vi "CalVEIN Main FRANK TEST.vi"() -> ()   [LabVIEW 2016]
uses:
  Type Defs/Sensor Data.ctl
  Type Defs/Boxcar.ctl
panel:
  out "1st loop":i32
  out "45% 2":string="31.00 °C"
  out "45%":string="31.10 °C"
  in  "Box cooler":bool
  out "NewVal":bool
  out "Ready To Fire Flag":bool
  out "Firing State":string[](array[string])=["System Is Not Armed", "", "", "", "", " "]
  in  "Arm Flag":bool
  in  "Sample Rate (secs)":u32=1000
  out "Burn Time\nCountdown (secs)":string="0.00"
  out "Boxcar Data":T1={"AI Sensor Data"={"Sensor Array"=[{"Description"="P2 - LOX Tank Pressure", "Last Reading"="-1.72", "Coefs"=[0.0, 5000.0], "Eng Units"="psig"}, {"Description"="P3 - Fuel Tank Pressure", "Last Reading"="-1.03", "Coefs"=[0.0, 5000.0], "Eng Units"="psig"}, {"Description"="P1 - Chamber Pressure", "Last Reading"="-1.17", "Coefs"=[0.0, 5000.0], "Eng Units"="psig"}, {"Description"="Not Used", "Last Reading"="0.00", "Coefs"=[0.0, 0.0], "Eng Units"="psig"}, {"Description"="P5- DOME Reg.", "Last Reading"="-1.58", "Coefs"=[0.0, 5000.0], "Eng Units"="psig"}, {"Description"="Not Use", "Last Reading"="0.00", "Coefs"=[0.0, 0.0], "Eng Units"="psig"}, {"Description"="P4- High Pressure Tank", "Last Reading"="-1.56", "Coefs"=[0.0, 10000.0], "Eng Units"="psig"}, {"Description"="P7 - Gnd High Pressure", "Last Reading"="-4.62", "Coefs"=[0.0, 10000.0], "Eng Units"="psig"}, {"Description"="P6 - GHE Fill Pressure", "Last Reading"="2.98", "Coefs"=[0.0, 5000.0], "Eng Units"="psig"}, {"Description"="P8 - Pneumatics Pressure", "Last Reading"="0.32", "Coefs"=[0.0, 5000.0], "Eng Units"="psig"}, {"Description"="Not Used", "Last Reading"="0.00", "Coefs"=[0.0, 0.0], "Eng Units"=""}, {"Description"="Not Used", "Last Reading"="0.00", "Coefs"=[0.0, 0.0], "Eng Units"=""}, {"Description"="Not Used", "Last Reading"="0.00", "Coefs"=[0.0, 0.0], "Eng Units"=""}, {"Description"="Not Used", "Last Reading"="0.00", "Coefs"=[0.0, 0.0], "Eng Units"=""}, {"Description"="Not Used", "Last Reading"="0.00", "Coefs"=[0.0, 0.0], "Eng Units"=""}, {"Description"="Not Used", "Last Reading"="0.00", "Coefs"=[0.0, 0.0], "Eng Units"=""}, {"Description"="QD Sep Indication", "Last Reading"="5.09", "Coefs"=[0.0, 1.0], "Eng Units"="On/Off"}, {"Description"="Lift Off Indicator", "Last Reading"="5.09", "Coefs"=[0.0, 1.0], "Eng Units"="On/Off"}, {"Description"="Main Valve Open Indicator", "Last Reading"="1.79", "Coefs"=[0.0, 1.0], "Eng Units"="On/Off"}, {"Description"="Main Valve Closed Indicator", "Last Reading"="1.76", "Coefs"=[0.0, 1.0], "Eng Units"="On/Off"}, {"Description"="Load Cell 1 - Veh Gross Weight", "Last Reading"="0.13", "Coefs"=[-122.0, 8333.3], "Eng Units"="lbf"}, {"Description"="Load Cell 2 - - Veh Gross Weight", "Last Reading"="-2.48", "Coefs"=[0.0, 8333.33], "Eng Units"="lbf"}, {"Description"="Not Used", "Last Reading"="0.00", "Coefs"=[0.0, 0.0], "Eng Units"=""}, {"Description"="Not Used", "Last Reading"="0.00", "Coefs"=[0.0, 0.0], "Eng Units"=""}, {"Description"="", "Last Reading"="0.00", "Coefs"=[], "Eng Units"=""}, {"Description"="", "Last Reading"="0.00", "Coefs"=[], "Eng Units"=""}, {"Description"="", "Last Reading"="0.00", "Coefs"=[], "Eng Units"=""}, {"Description"="", "Last Reading"="0.00", "Coefs"=[], "Eng Units"=""}, {"Description"="", "Last Reading"="0.00", "Coefs"=[], "Eng Units"=""}, {"Description"="", "Last Reading"="0.00", "Coefs"=[], "Eng Units"=""}, {"Description"="", "Last Reading"="0.00", "Coefs"=[], "Eng Units"=""}, {"Description"="", "Last Reading"="0.00", "Coefs"=[], "Eng Units"=""}]}, "TC Array"=[31.195067822, 31.09588569350001, 31.09588569350001, 30.99670356499999, 31.195067822, 31.09588569350001, 31.09588569350001, 1369.6815, 1369.6815, 1369.6815, 1369.6815, 1369.6815, 1369.6815, 1369.6815]}
  out "?":string="3.07 psig"
  out "Log Refnum":refnum<file>
  out "Log Epoch":u32
  out "Log Number":i32=123
  in  "Data Log Flag":bool
  out "File Path":path
  out "Eng Data & Units":string[](array[string])=["-1.67 psig", "-1.03 psig", "-1.17 psig", "0.00 psig", "-1.58 psig", "0.00 psig", "-1.56 psig", "-4.62 psig", "3.07 psig", "0.32 psig", "0.00 ", "0.00 ", "0.00 ", "0.00 ", "0.00 ", "0.00 ", "5.09 On/Off", "5.09 On/Off", "1.79 On/Off", "1.75 On/Off", "0.13 lbf", "-2.48 lbf", "0.00 ", "0.00 ", "0.00 ", "0.00 ", "0.00 ", "0.00 ", "0.00 ", "0.00 ", "0.00 ", "0.00 "]
  out "TC String Array":string[](array[string])=["31.20 °C", "31.10 °C", "31.10 °C", "31.00 °C", "31.20 °C", "31.10 °C", "31.10 °C", "1369.68 °C", "1369.68 °C", "1369.68 °C", "1369.68 °C", "1369.68 °C", "1369.68 °C", "1369.68 °C"]
  in  "Data Log Button":bool
  in  "Sequence Abort":bool
  out "Igniter Abort":bool
  out "Elapsed Time":u32=10554
  in  "Auto Sequence":bool
  in  "Auto Sequence Flag":bool
  out "Epoch":u32=5746771
  out "Countdown (secs)":i32
  in  "MV Open Start":dbl
  in  "Burn Time":dbl=3.0
  in  "Igniter Start":dbl=-3.0
  in  "Countdown":dbl=-10.0
  in  "Igniter Minimum\nTemp (°C)":dbl=200.0
  in  "Auto Switch":bool
  out "?":string="1369.68 °C"
  out "Thermometer 2":dbl(slide)=1369.6815 scale=0.0..1000.0
  out "Thermometer":dbl(slide)=1369.6815 scale=0.0..1000.0
  out "Igniter Temp (°C)":string="1369.68 °C"
  out "?":string="31.20 °C"
  out "30%":string="31.10 °C"
  out "QD Sep Indicator":bool=TRUE
  out "Liftoff Indicator":bool=TRUE
  out "MV Closed Ind":bool
  out "MV Open Ind":bool
  out "?":string="0.13 lbf"
  out "?":string="0.32 psig"
  out "?":string="-4.62 psig"
  out "?":string="-1.58 psig"
  out "?":string="-1.56 psig"
  out "?":string="-1.17 psig"
  out "P3":string="-1.03 psig"
  in  "High Press":bool
  in  "High Press Vent":bool
  in  "MV Open":bool
  in  "MV Closed":bool
  out "P2":string="-1.67 psig"
  in  "Remote QD Sep":bool
  in  "GHe Fill":bool
  in  "Igniter Pwr":bool
  in  "Dome Reg":bool
  in  "Dome Vent":bool
  in  "Fuel Vent":bool
  in  "LOX Vent":bool
  out "Relay States":bool[](array[boolean])
  in  "stop":bool
  in  "AI Sensor Data":T2={"Sensor Array"=[{"Description"="P2 - LOX Tank Pressure", "Last Reading"="-1.67", "Coefs"=[0.0, 5000.0], "Eng Units"="psig"}, {"Description"="P3 - Fuel Tank Pressure", "Last Reading"="-1.03", "Coefs"=[0.0, 5000.0], "Eng Units"="psig"}, {"Description"="P1 - Chamber Pressure", "Last Reading"="-1.17", "Coefs"=[0.0, 5000.0], "Eng Units"="psig"}, {"Description"="Not Used", "Last Reading"="0.00", "Coefs"=[0.0, 0.0], "Eng Units"="psig"}, {"Description"="P5- DOME Reg.", "Last Reading"="-1.58", "Coefs"=[0.0, 5000.0], "Eng Units"="psig"}, {"Description"="Not Use", "Last Reading"="0.00", "Coefs"=[0.0, 0.0], "Eng Units"="psig"}, {"Description"="P4- High Pressure Tank", "Last Reading"="-1.56", "Coefs"=[0.0, 10000.0], "Eng Units"="psig"}, {"Description"="P7 - Gnd High Pressure", "Last Reading"="-4.62", "Coefs"=[0.0, 10000.0], "Eng Units"="psig"}, {"Description"="P6 - GHE Fill Pressure", "Last Reading"="3.07", "Coefs"=[0.0, 5000.0], "Eng Units"="psig"}, {"Description"="P8 - Pneumatics Pressure", "Last Reading"="0.32", "Coefs"=[0.0, 5000.0], "Eng Units"="psig"}, {"Description"="Not Used", "Last Reading"="0.00", "Coefs"=[0.0, 0.0], "Eng Units"=""}, {"Description"="Not Used", "Last Reading"="0.00", "Coefs"=[0.0, 0.0], "Eng Units"=""}, {"Description"="Not Used", "Last Reading"="0.00", "Coefs"=[0.0, 0.0], "Eng Units"=""}, {"Description"="Not Used", "Last Reading"="0.00", "Coefs"=[0.0, 0.0], "Eng Units"=""}, {"Description"="Not Used", "Last Reading"="0.00", "Coefs"=[0.0, 0.0], "Eng Units"=""}, {"Description"="Not Used", "Last Reading"="0.00", "Coefs"=[0.0, 0.0], "Eng Units"=""}, {"Description"="QD Sep Indication", "Last Reading"="5.09", "Coefs"=[0.0, 1.0], "Eng Units"="On/Off"}, {"Description"="Lift Off Indicator", "Last Reading"="5.09", "Coefs"=[0.0, 1.0], "Eng Units"="On/Off"}, {"Description"="Main Valve Open Indicator", "Last Reading"="1.79", "Coefs"=[0.0, 1.0], "Eng Units"="On/Off"}, {"Description"="Main Valve Closed Indicator", "Last Reading"="1.75", "Coefs"=[0.0, 1.0], "Eng Units"="On/Off"}, {"Description"="Load Cell 1 - Veh Gross Weight", "Last Reading"="0.13", "Coefs"=[-122.0, 8333.3], "Eng Units"="lbf"}, {"Description"="Load Cell 2 - - Veh Gross Weight", "Last Reading"="-2.48", "Coefs"=[0.0, 8333.33], "Eng Units"="lbf"}, {"Description"="Not Used", "Last Reading"="0.00", "Coefs"=[0.0, 0.0], "Eng Units"=""}, {"Description"="Not Used", "Last Reading"="0.00", "Coefs"=[0.0, 0.0], "Eng Units"=""}, {"Description"="", "Last Reading"="0.00", "Coefs"=[], "Eng Units"=""}, {"Description"="", "Last Reading"="0.00", "Coefs"=[], "Eng Units"=""}, {"Description"="", "Last Reading"="0.00", "Coefs"=[], "Eng Units"=""}, {"Description"="", "Last Reading"="0.00", "Coefs"=[], "Eng Units"=""}, {"Description"="", "Last Reading"="0.00", "Coefs"=[], "Eng Units"=""}, {"Description"="", "Last Reading"="0.00", "Coefs"=[], "Eng Units"=""}, {"Description"="", "Last Reading"="0.00", "Coefs"=[], "Eng Units"=""}, {"Description"="", "Last Reading"="0.00", "Coefs"=[], "Eng Units"=""}]}
  # "CSULB Launch Team Control System"
  # "Questions regrads this system please direct them to Thanh Truc Le truclee126@gmail.com"
  # "Autosequence\n Parameters"
  # "30%"
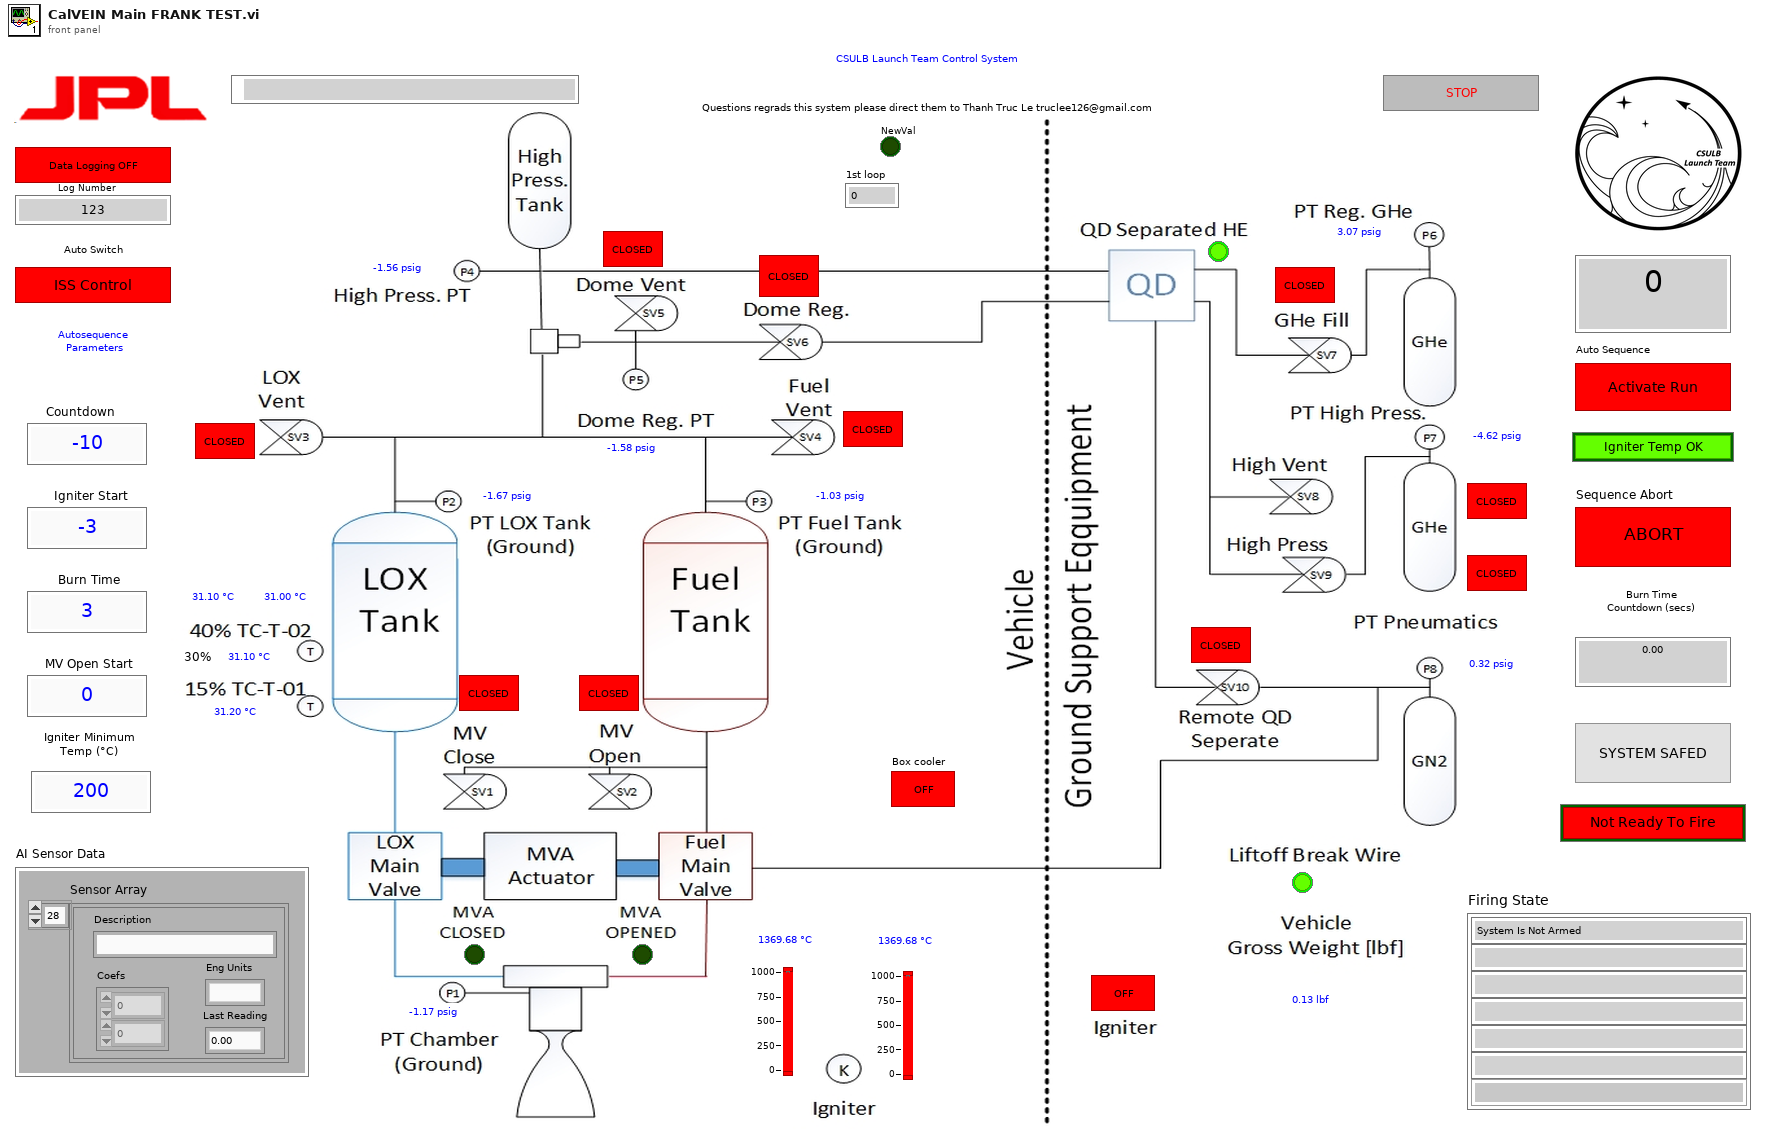
[diagram p1: front panel]
types:
  T1 = typedef "Boxcar.ctl" = cluster{"AI Sensor Data":T2, "TC Array":dbl[]}
  T2 = typedef "Sensor Data.ctl" = cluster{"Sensor Array":cluster{"Description":string, "Last Reading":string, "Coefs":dbl[], "Eng Units":string}[]}
  T3 = cluster{"Description":string, "Last Reading":string, "Coefs":dbl[], "Eng Units":string}[]
  T4 = enum16{"open", "replace", "create", "open or create", "replace or create", "replace or create with confirmation"}
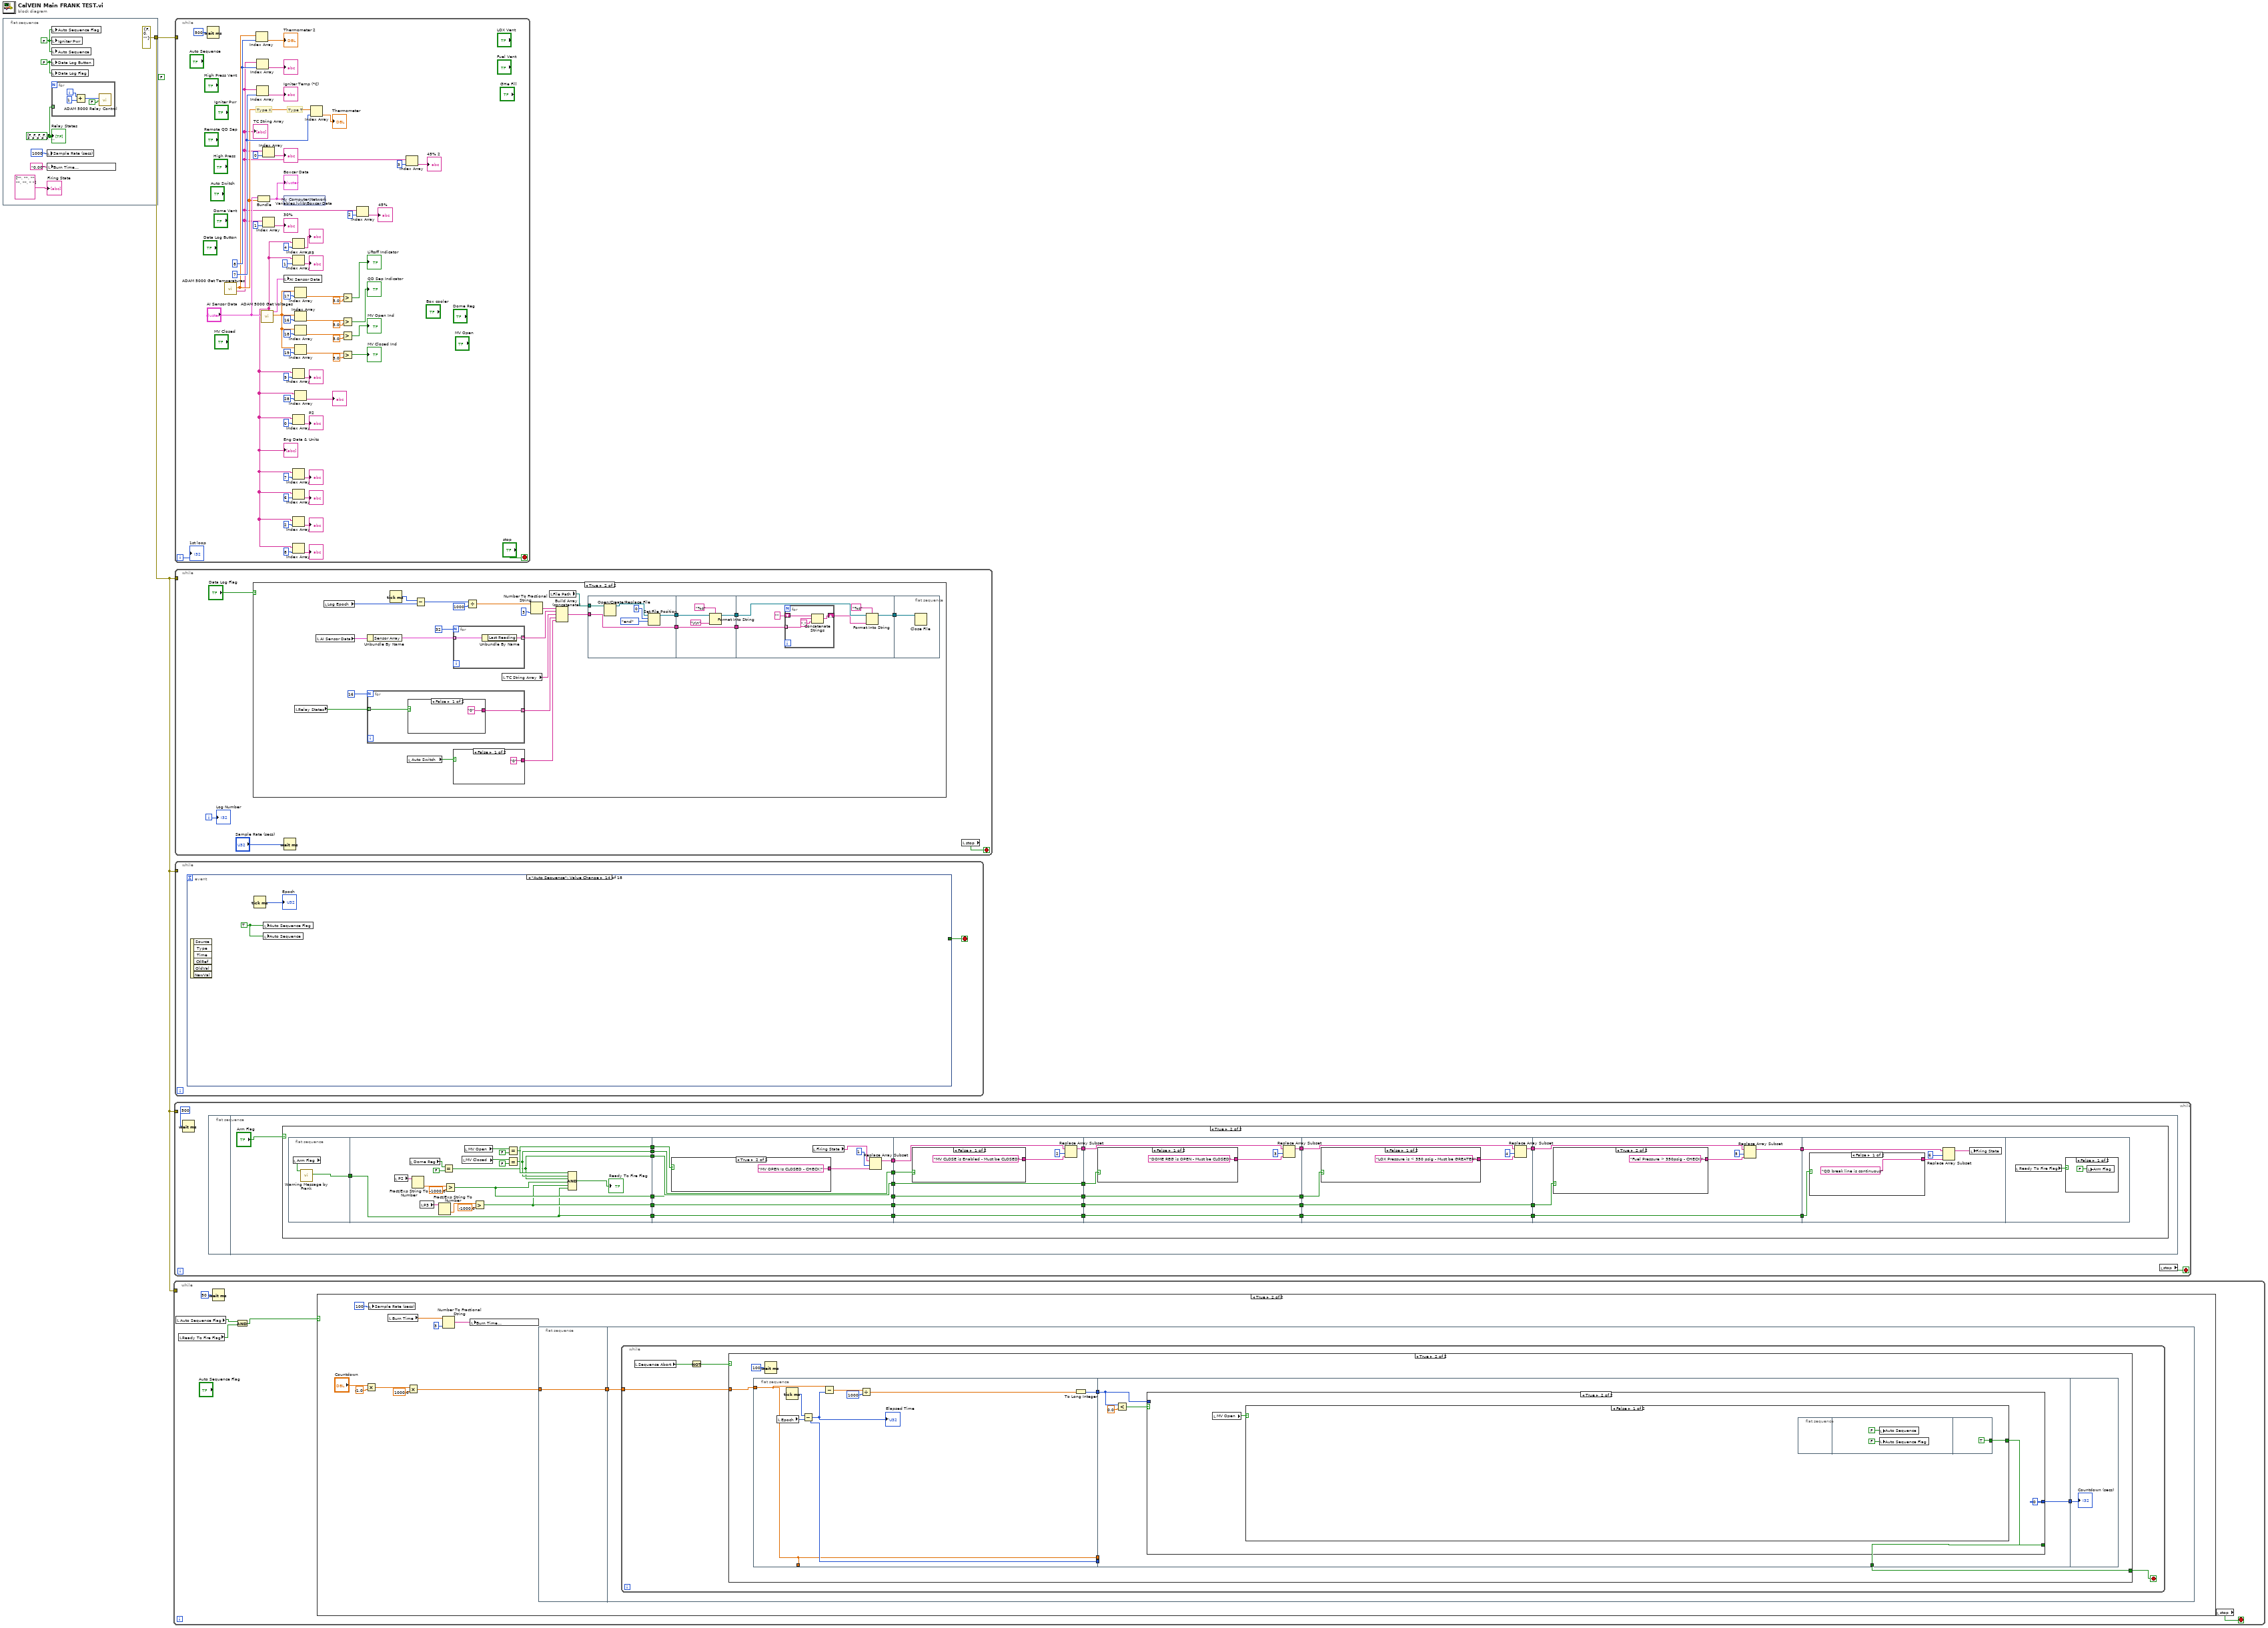
[diagram p0: block diagram]
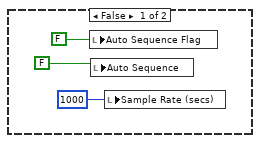
[diagram p2: hidden frame]
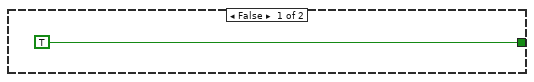
[diagram p3: hidden frame]
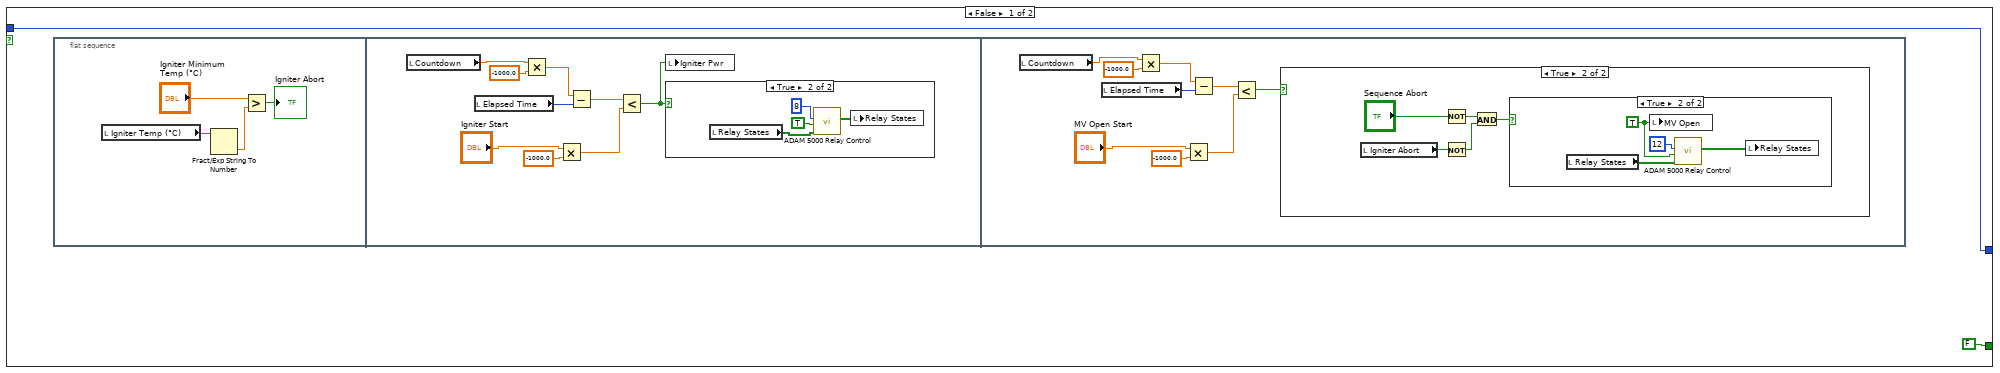
[diagram p4: hidden frame]
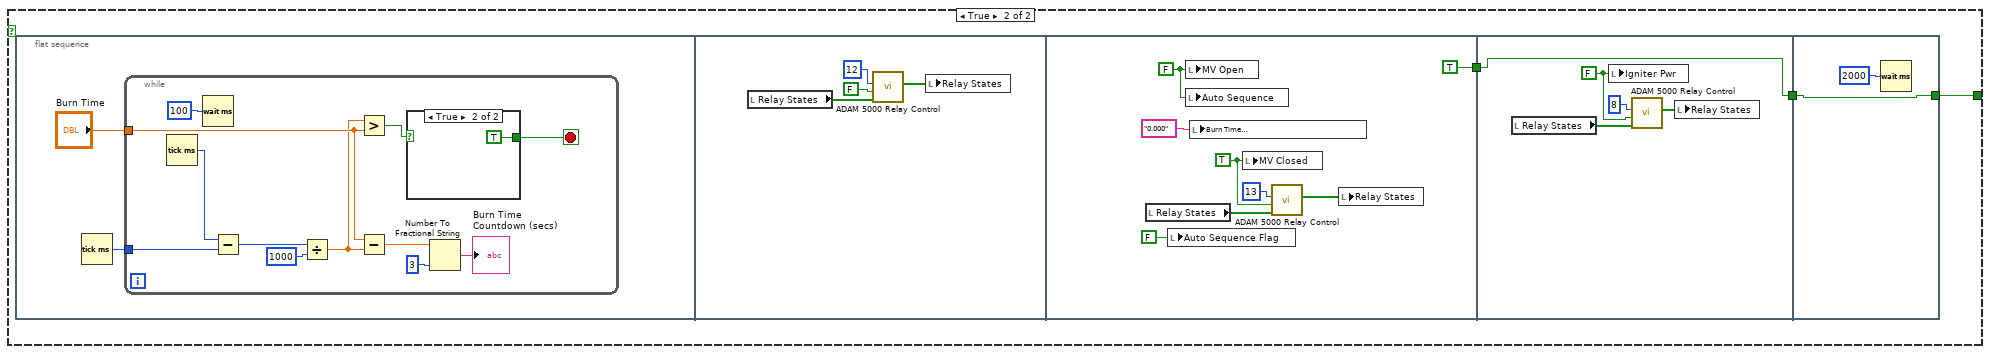
[diagram p8: hidden frame]
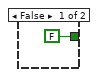
[diagram p9: hidden frame]
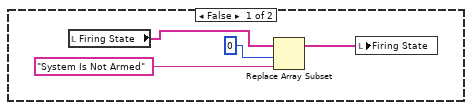
[diagram p10: hidden frame]
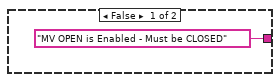
[diagram p11: hidden frame]
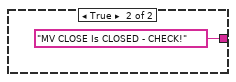
[diagram p12: hidden frame]
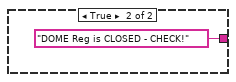
[diagram p13: hidden frame]
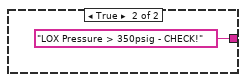
[diagram p14: hidden frame]
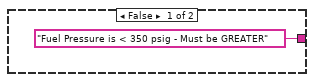
[diagram p15: hidden frame]
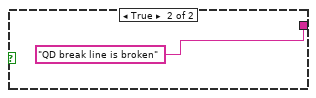
[diagram p16: hidden frame]
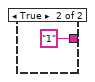
[diagram p19: hidden frame]
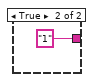
[diagram p20: hidden frame]
diagram:
  (unwired) FALSE
  n1 = flat-sequence {
    tunnel: [errorcluster {"status"=FALSE, "code"=0, "source"=""} ("error constant")] -> w1
    frame #0 {
      w5 = FALSE ("Data Lof Flag")
      w6 = FALSE ("Auto Sequence Flag")
      w7 = bool[] [FALSE, FALSE, FALSE, FALSE, FALSE, FALSE, FALSE, FALSE, FALSE, FALSE, FALSE, FALSE, FALSE, FALSE, FALSE, FALSE]
      n2 = local write "Sample Rate (secs)"(u32 1000 ("Sample Rate (secs)")) -> ()
      n3 = local write "Burn Time\nCountdown (secs)"("0.00" ("Burn Time\nCountdown (secs)")) -> ()
      n4 = local write "Auto Sequence Flag"(w6) -> ()
      n5 = local write "Igniter Pwr"(w6) -> ()
      n6 = local write "Auto Sequence"(w6) -> ()
      n7 = local write "Data Log Button"(w5) -> ()
      n8 = local write "Data Log Flag"(w5) -> ()
      n9 = for {
        tunnel: w7 -> [_] mode=indexing
        i -> [w12]
        n10 = Add(x=w12, y=1) -> (x+y=w10:i32)
        n11 = call "ADAM 5000 Relay Control.vi"("State"=FALSE, "Relay # (1=1st relay)"=w10) -> ()  [unwired: 9 in, 1 out]
      }
      "Relay States" <- w7
      "Firing State" <- string[] ["", "", "", "", "", " "]
    }
  }
  n12 = while {
    tunnel: w1 -> [_]
    stop <- w17 stop-if-true
    n13 = local read "Auto Sequence Flag"() -> (w14:bool)
    n14 = local read "Ready To Fire Flag"() -> (w15:bool)
    n15 = Wait (ms)(milliseconds to wait=u32 50) -> ()  [unwired: 1 out]
    n16 = And(x=w14, y=w15) -> (x .and. y?=w13:bool)
    n17 = case shown="True" w13 {
      frame False {
        n18 = local write "Auto Sequence Flag"(FALSE ("Auto Sequence Flag")) -> ()
        n19 = local write "Auto Sequence"(FALSE ("Auto Sequence Flag")) -> ()
        n20 = local write "Sample Rate (secs)"(u32 1000 ("Sample Rate (secs)")) -> ()
      }
      frame True {
        n21 = Multiply(x="Countdown", y=-1.0) -> (x*y=w25:dbl)
        n22 = local write "Sample Rate (secs)"(u32 100 ("Sample Rate (secs)")) -> ()
        n23 = local read "Burn Time"() -> (w24:dbl)
        n24 = Multiply(x=w25, y=1000.0) -> (x*y=w29:dbl)
        n25 = Number To Fractional String(number=w24, precision (6)=i16 3) -> (F-format string=w22:string)  [unwired: 2 in]
        n26 = local write "Burn Time\nCountdown (secs)"(w22) -> ()
        n27 = flat-sequence {
          tunnel: w29 -> [w31]
          tunnel: [w31] -> w28
          tunnel: w28 -> [w32]
          frame #0 {
          }
          frame #1 {
            n28 = while {
              tunnel: w32 -> [w36]
              stop <- w33 stop-if-true
              n29 = local read "Sequence Abort"() -> (w35:bool)
              n30 = Not(x=w35) -> (.not. x?=w34:bool)
              n31 = case shown="True" w34 {
                tunnel: w36 -> [_ w40]
                tunnel: [TRUE w38] -> w33
                frame False {
                }
                frame True {
                  n32 = flat-sequence {
                    tunnel: [w47] -> _
                    tunnel: w40 -> [w47]
                    tunnel: [w48] -> w44
                    tunnel: [w47] -> w43
                    tunnel: [w45] -> w42
                    tunnel: w44 -> [_]
                    tunnel: w43 -> [_]
                    tunnel: w42 -> [w54]
                    tunnel: [w56] -> w38
                    tunnel: [w53] -> w41
                    tunnel: w41 -> [w140]
                    frame #0 {
                      n33 = local read "Epoch"() -> (w46:u32)
                      n34 = Tick Count (ms)() -> (millisecond timer value=w52:u32)
                      n35 = Subtract(x=w52, y=w46) -> (x-y=w48:u32)
                      "Elapsed Time" <- w48
                      n36 = Subtract(x=w47, y=w48) -> (x-y=w49:dbl)
                      n37 = Divide(x=w49, y=u32 1000) -> (x/y=w50:dbl)
                      n38 = To Long Integer(number=w50) -> (32bit integer=w45:i32)
                    }
                    frame #1 {
                      n39 = Less?(x=w54, y=0.0) -> (x < y?=w55:bool)
                      n40 = case shown="True" w55 {
                        tunnel: [FALSE w97] -> w56
                        tunnel: w54 -> [w58 _]
                        tunnel: [w58 0] -> w53
                        frame False {
                          n41 = flat-sequence {
                            frame #0 {
                              n42 = local read "Igniter Temp (°C)"() -> (w63:string)
                              n43 = Fract/Exp String To Number(string=w63) -> (number=w62:dbl)  [unwired: 3 in, 1 out]
                              n44 = Greater?(x="Igniter Minimum\nTemp (°C)", y=w62) -> (0:→"Igniter Abort":bool)
                            }
                            frame #1 {
                              n45 = local read "Countdown"() -> (w72:dbl)
                              n46 = local read "Elapsed Time"() -> (w69:u32)
                              n47 = Multiply(x=w72, y=-1000.0) -> (x*y=w70:dbl)
                              n48 = Multiply(x="Igniter Start", y=-1000.0) -> (x*y=w65:dbl)
                              n49 = Subtract(x=w70, y=w69) -> (x-y=w66:dbl)
                              n50 = Less?(x=w66, y=w65) -> (x < y?=w64:bool)
                              n51 = local write "Igniter Pwr"(w64) -> ()
                              n52 = case shown="True" w64 {
                                frame False {
                                }
                                frame True {
                                n53 = local read "Relay States"() -> (w74:bool[])
                                n54 = call "ADAM 5000 Relay Control.vi"("Relay States IN"=w74, "State"=TRUE, "Relay # (1=1st relay)"=8) -> ("Relay States OUT"=w73:bool[])  [unwired: 8 in]
                                n55 = local write "Relay States"(w73) -> ()
                                }
                              }
                            }
                            frame #2 {
                              n56 = local read "Countdown"() -> (w79:dbl)
                              n57 = local read "Elapsed Time"() -> (w82:u32)
                              n58 = Multiply(x=w79, y=-1000.0) -> (x*y=w81:dbl)
                              n59 = Multiply(x="MV Open Start", y=-1000.0) -> (x*y=w85:dbl)
                              n60 = Subtract(x=w81, y=w82) -> (x-y=w84:dbl)
                              n61 = Less?(x=w84, y=w85) -> (x < y?=w77:bool)
                              n62 = case shown="True" w77 {
                                frame False {
                                }
                                frame True {
                                n63 = local read "Igniter Abort"() -> (w89:bool)
                                n64 = Not(x="Sequence Abort") -> (.not. x?=w88:bool)
                                n65 = Not(x=w89) -> (.not. x?=w87:bool)
                                n66 = And(x=w88, y=w87) -> (x .and. y?=w86:bool)
                                n67 = case shown="True" w86 {
                                frame False {
                                }
                                frame True {
                                w91 = TRUE ("State")
                                n68 = local read "Relay States"() -> (w93:bool[])
                                n69 = local write "MV Open"(w91) -> ()
                                n70 = call "ADAM 5000 Relay Control.vi"("Relay States IN"=w93, "State"=w91, "Relay # (1=1st relay)"=12) -> ("Relay States OUT"=w92:bool[])  [unwired: 8 in]
                                n71 = local write "Relay States"(w92) -> ()
                                }
                                }
                                }
                              }
                            }
                          }
                        }
                        frame True {
                          n72 = local read "MV Open"() -> (w95:bool)
                          n73 = case shown="False" w95 {
                            tunnel: [w98 w104] -> w97
                            frame False {
                              n74 = flat-sequence {
                                tunnel: [TRUE] -> w98
                                frame #0 {
                                }
                                frame #1 {
                                n75 = local write "Auto Sequence"(FALSE ("Auto Sequence Flag")) -> ()
                                n76 = local write "Auto Sequence Flag"(FALSE ("Auto Sequence Flag")) -> ()
                                }
                                frame #2 {
                                }
                              }
                            }
                            frame True {
                              n77 = flat-sequence {
                                tunnel: [TRUE] -> w103
                                tunnel: w103 -> [w137]
                                tunnel: [w137] -> w102
                                tunnel: [w139] -> w104
                                tunnel: w102 -> [w139]
                                frame #0 {
                                n78 = Tick Count (ms)() -> (millisecond timer value=w105:u32)
                                n79 = while {
                                tunnel: "Burn Time" -> [w111]
                                tunnel: w105 -> [w116]
                                stop <- w112 stop-if-true
                                n80 = Tick Count (ms)() -> (millisecond timer value=w117:u32)
                                n81 = Wait (ms)(milliseconds to wait=u32 100) -> ()  [unwired: 1 out]
                                n82 = Subtract(x=w117, y=w116) -> (x-y=w115:u32)
                                n83 = Divide(x=w115, y=u32 1000) -> (x/y=w110:dbl)
                                n84 = Greater?(x=w110, y=w111) -> (0:w113:bool)
                                n85 = Subtract(x=w111, y=w110) -> (x-y=w109:dbl)
                                n86 = case shown="True" w113 {
                                tunnel: [FALSE TRUE] -> w112
                                frame False {
                                }
                                frame True {
                                }
                                }
                                n87 = Number To Fractional String(number=w109, precision (6)=i16 3) -> (F-format string=→"Burn Time\nCountdown (secs)":string)  [unwired: 2 in]
                                }
                                }
                                frame #1 {
                                n88 = local read "Relay States"() -> (w123:bool[])
                                n89 = call "ADAM 5000 Relay Control.vi"("Relay States IN"=w123, "State"=FALSE, "Relay # (1=1st relay)"=12) -> ("Relay States OUT"=w124:bool[])  [unwired: 8 in]
                                n90 = local write "Relay States"(w124) -> ()
                                }
                                frame #2 {
                                w127 = FALSE ("Auto Sequence Flag")
                                w126 = TRUE ("State")
                                n91 = local read "Relay States"() -> (w130:bool[])
                                n92 = local write "Auto Sequence Flag"(FALSE ("Auto Sequence Flag")) -> ()
                                n93 = local write "MV Open"(w127) -> ()
                                n94 = local write "Auto Sequence"(w127) -> ()
                                n95 = local write "Burn Time\nCountdown (secs)"("0.000" ("Burn Time\nCountdown (secs)")) -> ()
                                n96 = local write "MV Closed"(w126) -> ()
                                n97 = call "ADAM 5000 Relay Control.vi"("Relay States IN"=w130, "State"=w126, "Relay # (1=1st relay)"=13) -> ("Relay States OUT"=w131:bool[])  [unwired: 8 in]
                                n98 = local write "Relay States"(w131) -> ()
                                }
                                frame #3 {
                                w133 = FALSE ("State")
                                n99 = local read "Relay States"() -> (w135:bool[])
                                n100 = local write "Igniter Pwr"(w133) -> ()
                                n101 = call "ADAM 5000 Relay Control.vi"("Relay States IN"=w135, "State"=w133, "Relay # (1=1st relay)"=8) -> ("Relay States OUT"=w134:bool[])  [unwired: 8 in]
                                n102 = local write "Relay States"(w134) -> ()
                                }
                                frame #4 {
                                n103 = Wait (ms)(milliseconds to wait=u32 2000) -> ()  [unwired: 1 out]
                                }
                              }
                            }
                          }
                        }
                      }
                    }
                    frame #2 {
                      "Countdown (secs)" <- w140
                    }
                  }
                  n104 = Wait (ms)(milliseconds to wait=u32 100) -> ()  [unwired: 1 out]
                }
              }
            }
          }
        }
      }
    }
    n105 = local read "stop"() -> (w17:bool)
  }
  n106 = while {
    tunnel: w1 -> [_]
    stop <- w141 stop-if-true
    n107 = Wait (ms)(milliseconds to wait=u32 500) -> ()  [unwired: 1 out]
    n108 = flat-sequence {
      frame #0 {
      }
      frame #1 {
        n109 = case shown="True" "Arm Flag" {
          frame False {
            n110 = local read "Firing State"() -> (w147:string[])
            n111 = Replace Array Subset(array=w147, new element="System Is Not Armed" ("new element/subarray"), index=0) -> (w144:string[])
            n112 = local write "Firing State"(w144) -> ()
          }
          frame True {
            n113 = flat-sequence {
              tunnel: [w176] -> w148
              tunnel: [w183] -> w174
              tunnel: [w182] -> w172
              tunnel: [w181] -> w168
              tunnel: [w180] -> w162
              tunnel: [w179] -> w157
              tunnel: [w177] -> w149
              tunnel: w148 -> [w177]
              tunnel: w174 -> [w205]
              tunnel: [w201] -> w173
              tunnel: w172 -> [w201]
              tunnel: [w200] -> w171
              tunnel: [w199] -> w169
              tunnel: w168 -> [w199]
              tunnel: [w198] -> w163
              tunnel: w162 -> [w198]
              tunnel: [w197] -> w158
              tunnel: w157 -> [w197]
              tunnel: [w196] -> w150
              tunnel: w149 -> [w196]
              tunnel: w173 -> [w214]
              tunnel: w171 -> [w213]
              tunnel: [w212] -> w170
              tunnel: w169 -> [w212]
              tunnel: [w211] -> w167
              tunnel: [w210] -> w164
              tunnel: w163 -> [w210]
              tunnel: [w209] -> w159
              tunnel: w158 -> [w209]
              tunnel: [w208] -> w151
              tunnel: w150 -> [w208]
              tunnel: w170 -> [w224]
              tunnel: w167 -> [w223]
              tunnel: [w222] -> w166
              tunnel: [w221] -> w165
              tunnel: w164 -> [w221]
              tunnel: [w220] -> w160
              tunnel: w159 -> [w220]
              tunnel: [w219] -> w152
              tunnel: w151 -> [w219]
              tunnel: w166 -> [w233]
              tunnel: w165 -> [w232]
              tunnel: [w231] -> w161
              tunnel: w160 -> [w231]
              tunnel: [w230] -> w156
              tunnel: [w229] -> w153
              tunnel: w152 -> [w229]
              tunnel: w161 -> [w241]
              tunnel: w156 -> [w240]
              tunnel: [w239] -> w155
              tunnel: [w238] -> w154
              tunnel: w153 -> [w238]
              tunnel: w155 -> [w248]
              tunnel: w154 -> [w246]
              frame #0 {
                n114 = local read "Arm Flag"() -> (w175:bool)
                n115 = call "Warning Message by Frank.vi"("Arm Flag"=w175) -> ("super ok"=w176:bool)  [unwired: 8 in, 2 out]
              }
              frame #1 {
                n116 = local read "P2"() -> (w189:string)
                n117 = local read "Dome Reg"() -> (w191:bool)
                n118 = Fract/Exp String To Number(string=w189) -> (number=w188:dbl)  [unwired: 3 in, 1 out]
                n119 = local read "P3"() -> (w184:string)
                n120 = Fract/Exp String To Number(string=w184) -> (number=w185:dbl)  [unwired: 3 in, 1 out]
                n121 = Equal?(x=w191, y=FALSE) -> (x = y?=w181:bool)
                n122 = Greater?(x=w188, y=-1000.0) -> (0:w180:bool)
                n123 = local read "MV Closed"() -> (w192:bool)
                n124 = local read "MV Open"() -> (w195:bool)
                n125 = Greater?(x=w185, y=-1000.0) -> (0:w179:bool)
                n126 = Equal?(x=w195, y=FALSE) -> (x = y?=w183:bool)
                n127 = Equal?(x=w192, y=FALSE) -> (x = y?=w182:bool)
                n128 = Compound Arithmetic op=AND(w183, w182, w181, w180, w179, w177) -> (→"Ready To Fire Flag":bool)
              }
              frame #2 {
                n129 = case shown="True" w205 {
                  tunnel: ["MV OPEN is Enabled - Must be CLOSED" "MV OPEN Is CLOSED - CHECK!"] -> w202
                  frame False {
                  }
                  frame True {
                  }
                }
                n130 = local read "Firing State"() -> (w204:string[])
                n131 = Replace Array Subset(array=w204, new element=w202, index=1) -> (w200:string[])
              }
              frame #3 {
                n132 = case shown="False" w214 {
                  tunnel: ["MV CLOSE is Enabled - Must be CLOSED" "MV CLOSE Is CLOSED - CHECK!"] -> w216
                  frame False {
                  }
                  frame True {
                  }
                }
                n133 = Replace Array Subset(array=w213, new element=w216, index=2) -> (w211:string[])
              }
              frame #4 {
                n134 = case shown="False" w224 {
                  tunnel: ["DOME REG is OPEN - Must be CLOSED" "DOME Reg is CLOSED - CHECK!"] -> w225
                  frame False {
                  }
                  frame True {
                  }
                }
                n135 = Replace Array Subset(array=w223, new element=w225, index=3) -> (w222:string[])
              }
              frame #5 {
                n136 = case shown="False" w232 {
                  tunnel: ["LOX Pressure is < 350 psig - Must be GREATER" "LOX Pressure > 350psig - CHECK!"] -> w235
                  frame False {
                  }
                  frame True {
                  }
                }
                n137 = Replace Array Subset(array=w233, new element=w235, index=4) -> (w230:string[])
              }
              frame #6 {
                n138 = case shown="True" w241 {
                  tunnel: ["Fuel Pressure is < 350 psig - Must be GREATER" "Fuel Pressure > 350psig - CHECK!"] -> w242
                  frame False {
                  }
                  frame True {
                  }
                }
                n139 = Replace Array Subset(array=w240, new element=w242, index=5) -> (w239:string[])
              }
              frame #7 {
                n140 = case shown="False" w246 {
                  tunnel: ["QD break line is continuous" "QD break line is broken"] -> w250
                  frame False {
                  }
                  frame True {
                  }
                }
                n141 = Replace Array Subset(array=w248, new element=w250, index=6) -> (w247:string[])
                n142 = local write "Firing State"(w247) -> ()
              }
              frame #8 {
                n143 = local read "Ready To Fire Flag"() -> (w253:bool)
                n144 = case shown="False" w253 {
                  frame False {
                    n145 = local write "Arm Flag"(FALSE ("Arm Flag")) -> ()
                  }
                  frame True {
                  }
                }
              }
            }
          }
        }
      }
    }
    n146 = local read "stop"() -> (w141:bool)
  }
  n147 = while {
    tunnel: w1 -> [_]
    i -> [w255]
    stop <- "stop" stop-if-true
    w268 = 8 ("index")
    w271 = 7 ("index")
    # "Type T"
    # "Type K"
    n148 = Wait (ms)(milliseconds to wait=u32 500) -> ()  [unwired: 1 out]
    n149 = call "ADAM 5000 Get Temperatures.vi"() -> ("TC String Array"=w257:string[], "TC Array"=w263:dbl[])  [unwired: 10 in]
    "TC String Array" <- w257
    n150 = Index Array(array=w263, index=w268) -> (element=→"Thermometer 2":dbl)
    n151 = Index Array(array=w257, index=w268) -> (element=→"?":string)
    n152 = Index Array(array=w257, index=w271) -> (element=→"Igniter Temp (°C)":string)
    n153 = Bundle("AI Sensor Data"="AI Sensor Data", "TC Array"=w263) -> (w262:cluster{"AI Sensor Data":T2, "TC Array":dbl[]})  [unwired: 1 in]
    "Boxcar Data" <- w262
    n154 = call "ADAM 5000 Get Voltages.vi"("AI Sensor Data"="AI Sensor Data") -> ("Master Raw Data Vdc"=w277:dbl[], "AI Sensor Data Out"=w310:T2, "Eng Data & Units"=w256:string[])  [unwired: 5 in, 3 out]
    "Eng Data & Units" <- w256
    n155 = Index Array(array=w257, index=0) -> (element=→"?":string)
    n156 = Index Array(array=w257, index=1) -> (element=→"30%":string)
    n157 = shared-variable "My Computer\\Network Variables.lvlib\\Boxcar Data"(w262) -> ()  [unwired: 1 in, 1 out]
    n158 = local write "AI Sensor Data"(w310) -> ()
    n159 = Index Array(array=w256, index=4) -> (element=→"?":string)
    n160 = Index Array(array=w256, index=1) -> (element=→"P3":string)
    n161 = Index Array(array=w256, index=9) -> (element=→"?":string)
    n162 = Index Array(array=w256, index=0) -> (element=→"P2":string)
    n163 = Index Array(array=w256, index=7) -> (element=→"?":string)
    n164 = Index Array(array=w256, index=6) -> (element=→"?":string)
    n165 = Index Array(array=w256, index=2) -> (element=→"?":string)
    n166 = Index Array(array=w256, index=8) -> (element=→"?":string)
    n167 = Index Array(array=w277, index=17) -> (element=w284:dbl)
    n168 = Index Array(array=w277, index=16) -> (element=w279:dbl)
    n169 = Index Array(array=w277, index=18) -> (element=w292:dbl)
    n170 = Index Array(array=w277, index=19) -> (element=w288:dbl)
    n171 = Index Array(array=w256, index=28) -> (element=→"?":string)
    n172 = Index Array(array=w263, index=w271) -> (element=→"Thermometer":dbl)
    n173 = Greater?(x=w284, y=3.0) -> (0:→"Liftoff Indicator":bool)
    n174 = Greater?(x=w279, y=3.0) -> (0:→"QD Sep Indicator":bool)
    n175 = Greater?(x=w292, y=3.0) -> (0:→"MV Open Ind":bool)
    n176 = Greater?(x=w288, y=3.0) -> (0:→"MV Closed Ind":bool)
    n177 = Index Array(array=w257, index=2) -> (element=→"45%":string)
    n178 = Index Array(array=w257, index=3) -> (element=→"45% 2":string)
    "1st loop" <- w255
  }
  n179 = while {
    tunnel: w1 -> [_]
    i -> [w314]
    stop <- w316 stop-if-true
    n180 = case shown="True" "Data Log Flag" {
      frame False {
      }
      frame True {
        n181 = local read "Relay States"() -> (w338:bool[])
        n182 = local read "AI Sensor Data"() -> (w340:T2)
        n183 = local read "Log Epoch"() -> (w331:u32)
        n184 = Unbundle By Name(w340) -> ("Sensor Array"=w339:T3)
        n185 = for {
          N: 16 -> [_]
          tunnel: w338 -> [w366] mode=indexing
          tunnel: [w365] -> w334 mode=indexing
          n186 = case shown="False" w366 {
            tunnel: ["0" "1"] -> w365
            frame False {
            }
            frame True {
            }
          }
        }
        n187 = Tick Count (ms)() -> (millisecond timer value=w332:u32)
        n188 = local read "Auto Switch"() -> (w337:bool)
        n189 = Subtract(x=w332, y=w331) -> (x-y=w330:u32)
        n190 = for {
          N: 32 -> [_]
          tunnel: w339 -> [w370] mode=indexing
          tunnel: [w369] -> w336 mode=indexing
          n191 = Unbundle By Name(w370) -> ("Last Reading"=w369:string)
        }
        n192 = case shown="False" w337 {
          tunnel: ["0" "1"] -> w333
          frame False {
          }
          frame True {
          }
        }
        n193 = Divide(x=w330, y=u32 1000) -> (x/y=w328:dbl)
        n194 = local read "TC String Array"() -> (w335:string[])
        n195 = Number To Fractional String(number=w328, precision (6)=i16 3) -> (F-format string=w326:string)  [unwired: 2 in]
        n196 = local read "File Path"() -> (w325:path)
        n197 = Build Array (concatenate)(w326, w336, w335, w334, w333) -> (w324:string[])
        n198 = flat-sequence {
          tunnel: w324 -> [w346]
          tunnel: w325 -> [w345]
          tunnel: [w346] -> w322
          tunnel: [w341] -> w319
          tunnel: [w347] -> w323
          tunnel: w322 -> [w351]
          tunnel: [w351] -> w321
          tunnel: w319 -> [w348]
          tunnel: w323 -> [w354]
          tunnel: w321 -> [w357]
          tunnel: [w352] -> w320
          tunnel: w320 -> [w362]
          frame #0 {
            n199 = Open/Create/Replace File(file path (use dialog)=w345) -> (refnum out=w344:refnum<file>)  [unwired: 5 in, 2 out]
            n200 = Set File Position(offset (in bytes) (0)=i64 0, refnum=w344, from (0:start)=enum16{"start", "end", "current"}."end") -> (refnum out=w341:refnum<file>)  [unwired: 1 in, 1 out]
          }
          frame #1 {
            n201 = Format Into String(format string="%s", initial string=w348, "\r\n") -> (resulting string=w347:refnum<file>)  [unwired: 1 in, 1 out]
          }
          frame #2 {
            n202 = for {
              shift-right: [w359] -> w353
              shift-left: "" -> [w358]
              tunnel: w357 -> [w361] mode=indexing
              n203 = Concatenate Strings(w358, w361, "," ("string")) -> (w359:string)
            }
            n204 = Format Into String(format string="%s", initial string=w354, w353) -> (resulting string=w352:refnum<file>)  [unwired: 1 in, 1 out]
          }
          frame #3 {
            n205 = Close File(refnum=w362) -> ()  [unwired: 1 in, 2 out]
          }
        }
      }
    }
    n206 = Wait (ms)(milliseconds to wait="Sample Rate (secs)") -> ()  [unwired: 1 out]
    n207 = local read "stop"() -> (w316:bool)
    "Log Number" <- w314
  }
  n208 = while {
    tunnel: w1 -> [_]
    stop <- w371 stop-if-true
    n209 = event shown="[13] \"Auto Sequence\": Value Change" {
      selector: _ -> [_ _ _ _ _ _ _ _ _ _ _ _ _ _ _ _ _ _]
      dyn-events: _ -> [_ _ _ _ _ _ _ _ _ _ _ _ _ _ _ _ _ _]
      timeout: _ -> [_ _ _ _ _ _ _ _ _ _ _ _ _ _ _ _ _ _]
      tunnel: [_ _ _ _ _ _ _ _ w400 _ _ _ _ _ _ _ _ _] -> w371
      event Timeout {
        n210 = event-data() -> ()  [unwired: 1 in, 3 out]
      }
      event "LOX Vent": Value Change {
        n211 = event-data() -> ("NewVal"=w374:bool)  [unwired: 1 in, 5 out]
        n212 = local read "Relay States"() -> (w373:bool[])
        n213 = call "ADAM 5000 Relay Control.vi"("Relay States IN"=w373, "State"=w374, "Relay # (1=1st relay)"=1) -> ("Relay States OUT"=w372:bool[])  [unwired: 8 in]
        n214 = local write "Relay States"(w372) -> ()
      }
      event "Fuel Vent": Value Change {
        n215 = event-data() -> ("NewVal"=w376:bool)  [unwired: 1 in, 5 out]
        n216 = local read "Relay States"() -> (w378:bool[])
        n217 = call "ADAM 5000 Relay Control.vi"("Relay States IN"=w378, "State"=w376, "Relay # (1=1st relay)"=2) -> ("Relay States OUT"=w377:bool[])  [unwired: 8 in]
        n218 = local write "Relay States"(w377) -> ()
      }
      event "Dome Vent": Value Change {
        n219 = event-data() -> ("NewVal"=w380:bool)  [unwired: 1 in, 5 out]
        n220 = local read "Relay States"() -> (w382:bool[])
        n221 = call "ADAM 5000 Relay Control.vi"("Relay States IN"=w382, "State"=w380, "Relay # (1=1st relay)"=6) -> ("Relay States OUT"=w381:bool[])  [unwired: 8 in]
        n222 = local write "Relay States"(w381) -> ()
      }
      event "Dome Reg": Value Change {
        n223 = event-data() -> ("NewVal"=w384:bool)  [unwired: 1 in, 5 out]
        n224 = local read "Relay States"() -> (w386:bool[])
        n225 = call "ADAM 5000 Relay Control.vi"("Relay States IN"=w386, "State"=w384, "Relay # (1=1st relay)"=5) -> ("Relay States OUT"=w385:bool[])  [unwired: 8 in]
        n226 = local write "Relay States"(w385) -> ()
      }
      event "Igniter Pwr": Value Change {
        n227 = event-data() -> ("NewVal"=w388:bool)  [unwired: 1 in, 5 out]
        n228 = local read "Relay States"() -> (w390:bool[])
        n229 = call "ADAM 5000 Relay Control.vi"("Relay States IN"=w390, "State"=w388, "Relay # (1=1st relay)"=8) -> ("Relay States OUT"=w389:bool[])  [unwired: 8 in]
        n230 = local write "Relay States"(w389) -> ()
      }
      event "GHe Fill": Value Change {
        n231 = event-data() -> ("NewVal"=w392:bool)  [unwired: 1 in, 5 out]
        n232 = local read "Relay States"() -> (w394:bool[])
        n233 = call "ADAM 5000 Relay Control.vi"("Relay States IN"=w394, "State"=w392, "Relay # (1=1st relay)"=9) -> ("Relay States OUT"=w393:bool[])  [unwired: 8 in]
        n234 = local write "Relay States"(w393) -> ()
      }
      event "Remote QD Sep": Value Change {
        n235 = event-data() -> ("NewVal"=w396:bool)  [unwired: 1 in, 5 out]
        n236 = local read "Relay States"() -> (w398:bool[])
        n237 = call "ADAM 5000 Relay Control.vi"("Relay States IN"=w398, "State"=w396, "Relay # (1=1st relay)"=10) -> ("Relay States OUT"=w397:bool[])  [unwired: 8 in]
        n238 = local write "Relay States"(w397) -> ()
      }
      event "stop": Value Change {
        n239 = event-data() -> ()  [unwired: 1 in, 6 out]
        n240 = flat-sequence {
          tunnel: [TRUE] -> w400
          frame #0 {
            n241 = Wait (ms)(milliseconds to wait=u32 2000) -> ()  [unwired: 1 out]
          }
          frame #1 {
          }
        }
      }
      event "MV Closed": Value Change {
        n242 = event-data() -> ("NewVal"=w403:bool)  [unwired: 1 in, 5 out]
        n243 = local read "Relay States"() -> (w405:bool[])
        n244 = call "ADAM 5000 Relay Control.vi"("Relay States IN"=w405, "State"=w403, "Relay # (1=1st relay)"=13) -> ("Relay States OUT"=w404:bool[])  [unwired: 8 in]
        n245 = local write "Relay States"(w404) -> ()
      }
      event "High Press Vent": Value Change {
        n246 = event-data() -> ("NewVal"=w407:bool)  [unwired: 1 in, 5 out]
        n247 = local read "Relay States"() -> (w409:bool[])
        n248 = call "ADAM 5000 Relay Control.vi"("Relay States IN"=w409, "State"=w407, "Relay # (1=1st relay)"=15) -> ("Relay States OUT"=w408:bool[])  [unwired: 8 in]
        n249 = local write "Relay States"(w408) -> ()
      }
      event "High Press": Value Change {
        n250 = event-data() -> ("NewVal"=w411:bool)  [unwired: 1 in, 5 out]
        n251 = local read "Relay States"() -> (w413:bool[])
        n252 = call "ADAM 5000 Relay Control.vi"("Relay States IN"=w413, "State"=w411, "Relay # (1=1st relay)"=7) -> ("Relay States OUT"=w412:bool[])  [unwired: 8 in]
        n253 = local write "Relay States"(w412) -> ()
      }
      event "Auto Switch": Value Change {
        n254 = event-data() -> ("NewVal"=w416:bool)  [unwired: 1 in, 5 out]
        n255 = call "Control ETH008 Relay.vi"("On/Off"=w416, "Relay Number"=1) -> ()  [unwired: 10 in]
      }
      event "Auto Sequence": Value Change {
        w418 = TRUE ("Auto Sequence Flag")
        n256 = event-data() -> ()  [unwired: 1 in, 6 out]
        n257 = Tick Count (ms)() -> (millisecond timer value=→"Epoch":u32)
        n258 = local write "Auto Sequence Flag"(w418) -> ()
        n259 = local write "Auto Sequence"(w418) -> ()
      }
      event "Sequence Abort": Value Change {
        n260 = event-data() -> ()  [unwired: 1 in, 6 out]
        n261 = flat-sequence {
          frame #0 {
            w419 = FALSE ("Auto Sequence Flag")
            n262 = local write "Auto Sequence Flag"(w419) -> ()
            n263 = local write "Igniter Pwr"(w419) -> ()
            n264 = local write "Auto Sequence"(w419) -> ()
          }
          frame #1 {
            n265 = for {
              tunnel: bool[] [FALSE, FALSE, FALSE, FALSE, FALSE, FALSE, FALSE, FALSE, FALSE, FALSE, FALSE, FALSE, FALSE, FALSE, FALSE, FALSE] -> [_] mode=indexing
              i -> [w424]
              n266 = Add(x=w424, y=1) -> (x+y=w422:i32)
              n267 = call "ADAM 5000 Relay Control.vi"("State"=FALSE, "Relay # (1=1st relay)"=w422) -> ()  [unwired: 9 in, 1 out]
            }
          }
        }
      }
      event "Data Log Button": Value Change {
        n268 = event-data() -> ("NewVal"=w425:bool)  [unwired: 1 in, 5 out]
        n269 = case shown="True" w425 {
          frame False {
            n270 = local write "Data Log Flag"(FALSE ("Data Lof Flag")) -> ()
            n271 = local write "Data Log Flag"(FALSE ("Data Lof Flag")) -> ()
            n272 = local write "Data Log Flag"(FALSE ("Data Lof Flag")) -> ()
            n273 = local write "Data Log Flag"(FALSE ("Data Lof Flag")) -> ()
            n274 = local write "Data Log Flag"(FALSE ("Data Lof Flag")) -> ()
            n275 = local write "Data Log Flag"(FALSE ("Data Lof Flag")) -> ()
            n276 = local write "Data Log Flag"(FALSE ("Data Lof Flag")) -> ()
            n277 = local write "Data Log Flag"(FALSE ("Data Lof Flag")) -> ()
            n278 = local write "Data Log Flag"(FALSE ("Data Lof Flag")) -> ()
            n279 = local write "Data Log Flag"(FALSE ("Data Lof Flag")) -> ()
            n280 = local write "Data Log Flag"(FALSE ("Data Lof Flag")) -> ()
          }
          frame True {
            n281 = flat-sequence {
              frame #0 {
                n282 = Tick Count (ms)() -> (millisecond timer value=→"Log Epoch":u32)
                n283 = for {
                  N: 14 -> [_]
                  tunnel: [w469] -> w448 mode=indexing
                  i -> [w468]
                  n284 = Add(x=w468, y=1) -> (x+y=w466:i32)
                  n285 = Number To Fractional String(number=w466, precision (6)=i16 0) -> (F-format string=w470:string)  [unwired: 2 in]
                  n286 = Concatenate Strings("TC", w470) -> (w469:string)
                }
                n287 = for {
                  N: 16 -> [_]
                  tunnel: [w462] -> w447 mode=indexing
                  i -> [w461]
                  n288 = Add(x=w461, y=1) -> (x+y=w459:i32)
                  n289 = Number To Fractional String(number=w459, precision (6)=i16 0) -> (F-format string=w463:string)  [unwired: 2 in]
                  n290 = Concatenate Strings("Relay", w463) -> (w462:string)
                }
                n291 = local read "AI Sensor Data"() -> (w454:T2)
                n292 = Unbundle By Name(w454) -> ("Sensor Array"=w453:T3)
                n293 = for {
                  tunnel: w453 -> [w474] mode=indexing
                  tunnel: [w473] -> w451 mode=indexing
                  n294 = Unbundle By Name(w474) -> ("Description"=w473:string)
                }
                n295 = Build Array (concatenate)("Time (s)", w451, w448, w447, "Manual/Auto (1=Auto)") -> (w443:string[])
                n296 = for {
                  shift-right: [w456] -> w441
                  shift-left: "" -> [w455]
                  tunnel: w443 -> [w458] mode=indexing
                  n297 = Concatenate Strings(w455, w458, "," ("string")) -> (w456:string)
                }
                n298 = Open/Create/Replace File(operation (0:open)=T4."replace or create") -> (refnum out=w440:refnum<file>)  [unwired: 5 in, 2 out]
                "Log Refnum" <- w440
                n299 = Refnum to Path(1:w440) -> (0:→"File Path":path)
                n300 = Format Into String(format string="%s", initial string=w440, w441) -> (resulting string=w437:refnum<file>)  [unwired: 1 in, 1 out]
                n301 = Close File(refnum=w437) -> ()  [unwired: 1 in, 2 out]
              }
              frame #1 {
                n302 = Wait (ms)(milliseconds to wait=u32 1000) -> ()  [unwired: 1 out]
              }
              frame #2 {
                n303 = local write "Data Log Flag"(TRUE ("Data Lof Flag")) -> ()
              }
            }
          }
        }
      }
      event "MV Open": Value Change {
        n304 = event-data() -> ("NewVal"=w480:bool)  [unwired: 1 in, 5 out]
        "NewVal" <- w480
        n305 = local read "Relay States"() -> (w478:bool[])
        n306 = call "ADAM 5000 Relay Control.vi"("Relay States IN"=w478, "State"=w480, "Relay # (1=1st relay)"=12) -> ("Relay States OUT"=w479:bool[])  [unwired: 8 in]
        n307 = local write "Relay States"(w479) -> ()
      }
      event "Box cooler": Value Change {
        n308 = event-data() -> ("NewVal"=w481:bool)  [unwired: 1 in, 5 out]
        n309 = local read "Relay States"() -> (w483:bool[])
        n310 = call "ADAM 5000 Relay Control.vi"("Relay States IN"=w483, "State"=w481, "Relay # (1=1st relay)"=3) -> ("Relay States OUT"=w484:bool[])  [unwired: 8 in]
        n311 = local write "Relay States"(w484) -> ()
      }
    }
  }
